vi "Test Executive.vi"(11 "Module Config":T30={"Name"="Test Executive", "Parent Q"=refnum, "Is Child?"=FALSE, "Index"=0, "Dirs"={"Root"=path "C:/MTE", "Config"=path "C:/MTE/Config", "Logs"=path "C:/MTE/Logs", "Reports"=path "C:/ATE/Reports", "App Data"=path "C:/ProgramData/Test Executive"}, "Simulate"=FALSE, "SimCtrl"=refnum}) -> ()   [LabVIEW 2018] (continued)
                  n74 = To More Generic Class(target class=w219, reference=w220) -> (generic class reference=w218:refnum<vi>)
                  n75 = To More Generic Class(target class=w219, reference=w223) -> (generic class reference=w224:refnum<vi>)
                  n76 = To More Generic Class(target class=w219, reference=w221) -> (generic class reference=w222:refnum<vi>)
                  n77 = Build Array (concatenate)(w225, w224, w222, w218) -> (w226:refnum<vi>[])
                }
                frame 99, Default {
                  # "Done"
                }
              }
            }
            n78 = Unbundle By Name(w208) -> ("CtrlStates"=w210:refnum<class "Class.SaveCtrls.lvclass">, "Cfg.Name"=w212:string, "Cfg.Dirs.App Data"=w211:path)
            n79 = call-dynamic "Class.SaveCtrls.InitLoadRestore.vi"("Ctrl Array"=w209, "Module Data Dir"=w211, "Module Name"=w212, "CtrlStates In"=w210) -> ("CtrlStates"=w207:refnum<class "Class.SaveCtrls.lvclass">)  [unwired: 6 in, 1 out]
          }
          frame #5 {
            w229 = T17[] []  # RptCfg
            w230 = T58[] []  # Subscr
            w232 = FALSE  # TestCanceled
            w233 = T20 {"DispDetails"=FALSE, "NotResetSN"=FALSE, "NotValOper"=FALSE, "NotValSN"=FALSE, "DisResults"=FALSE, "StaModule"=FALSE, "EditEQ"=FALSE, "ClrWarn"=FALSE, "ClrErr"=FALSE, "ViewCfg"=FALSE, "SetOpts"=FALSE, "ContOnErr"=FALSE, "ContOnFail"=FALSE, "DisMetrics"=FALSE, "SelSeq"=FALSE, "GenRpt"=FALSE, "DisStartWithSN"=FALSE, "Auto Repeat Seq En"=FALSE, "DataDirEn"=FALSE, "SNRouteCk"=FALSE}  # Opts
            w238 = path ""  # UUT Dir
            w239 = -1.0  # Repeat(s)
            w241 = T69 {"Limits"=variant, "Limit File"="", "Limit Ver"="", "RsltCodes"=variant, "Rslt Code File"="", "Rslt Code Ver"="", "Default Seq"=0, "FaultPrefix"=0, "UUTRoutes"=[], "DisableRouteCk"=FALSE, "StaVer"=0, "SN Valid"=FALSE, "ReqVars"=FALSE, "Product"="", "ProcessStep"="", "FileSyncMaster"=path "", "CmtPrmpt"=FALSE}  # Lists
            w243 = T50 {"Position"="", "Result"={"Result"=enum."Pass", "Code"=0, "Description"=""}, "Measurements"={"Measurement"=[]}, "UUTInfo"={"Product"="", "Desc"="", "PN"="", "SN"="", "Lot"="", "DateCode"="", "AltID"="", "Revision"="", "Properties"={"Property"=[]}}}  # RptUUT
            w242 = T70 {"#attributes"={"Version"="MTE_2.0.0"}, "Facility"={"Name"="", "Location"=""}, "Station"={"Name"="", "PN"="", "SN"="", "Rev"="", "PC Name"="", "Location"="", "HW_Config"={"HW_Item"=[]}, "SW_Config"={"SW_Item"=[]}}, "Test Run"={"Operator"="", "Start Time"=timestamp(0 s since 1904-01-01), "Duration(s)"=0.0, "Mode"="", "Comment"="", "ProcessStep"=""}, "Test Sequence"={"Name"="", "Config"={"Config_Item"=[]}}}  # RptHdr
            w244 = cluster{"FileObjs":T29[], "Meas":T38[]} {"FileObjs"=[], "Meas"=[{"Cnt"=0, "Step"="", "Category"="", "Name"="", "Value"="", "Units"="", "LimType"="", "LL"="", "UL"="", "Status"=0, "Code"=0, "Desc"="", "Time"=timestamp(0 s since 1904-01-01)}]}  # Data
            w245 = T72 {"Level"=0, "Cnts"=[], "Step"="", "Cntr"=0}  # SectCtr
            w246 = errorcluster {"status"=FALSE, "code"=0, "source"=""}  # ResultError
            w247 = FALSE  # DisableResults
            w231 = variant  # SW_Vers
            n80 = call <vilib>:"Q.Enqueue Task.vi"("Top of Q"=TRUE, "Task Name"="Test Metrics - Load", "Q In"=w236) -> ("Q Out"=w237:refnum<queue>)  [unwired: 7 in, 1 out]
            n81 = call <vilib>:"Q.Enqueue Seq.vi"("Top of Q"=TRUE, "Seq Task Name"="Init Controls", "Q In"=w237) -> ()  [unwired: 7 in, 2 out]
            "Failing Status" <- "Failing" ("Failing Status")
          }
          frame #6 {
            # "Setup Menu"
            n82 = Current VI's Menubar() -> (w250:refnum<k9>)
            n83 = while {
              tunnel: w250 -> [w251]
              i -> [w253]
              stop <- w252 stop-if-true
              n84 = case shown="1" w253 {
                tunnel: [_ _ _ _ _ _ _ _ _ _ TRUE] -> w252
                tunnel: w251 -> [w259 w260 w265 w268 w271 w274 w277 w280 w284 w288 w290]
                frame 0 {
                  w256 = "Data"
                  n85 = Insert Menu Items(4:"Config" ("menu tag"), 7:w256, 8:w256, 9:w259) -> (0:w254:errorcluster, 3:w257:refnum<k9>)  [unwired: 2 in, 1 out]
                  n86 = call <vilib>:"Menu.Enable Item.vi"("error in"=w254, "Enable"=FALSE, "Tag"=w256, "Menu Ref"=w257) -> ()  [unwired: 6 in, 2 out]
                }
                frame 1 {
                  w262 = "Route Check"
                  n87 = Insert Menu Items(4:"Config" ("menu tag"), 7:w262, 8:w262, 9:w260) -> ()  [unwired: 2 in, 3 out]
                }
                frame 2 {
                  w264 = "Test Executive"
                  n88 = Insert Menu Items(5:"Config" ("menu tag"), 7:w264, 8:w264, 9:w265) -> ()  [unwired: 2 in, 3 out]
                }
                frame 3 {
                  w267 = "Local Station"
                  n89 = Insert Menu Items(5:"Config" ("menu tag"), 7:w267, 8:w267, 9:w268) -> ()  [unwired: 2 in, 3 out]
                }
                frame 4 {
                  w270 = "File Sync"
                  n90 = Insert Menu Items(5:"Config" ("menu tag"), 7:w270, 8:w270, 9:w271) -> ()  [unwired: 2 in, 3 out]
                }
                frame 5 {
                  w273 = "File Rotate"
                  n91 = Insert Menu Items(5:"Config" ("menu tag"), 7:w273, 8:w273, 9:w274) -> ()  [unwired: 2 in, 3 out]
                }
                frame 6 {
                  w276 = "Test Reports"
                  n92 = Insert Menu Items(5:"Config" ("menu tag"), 7:w276, 8:w276, 9:w277) -> ()  [unwired: 2 in, 3 out]
                }
                frame 7 {
                  w279 = "Mode Manager"
                  n93 = Insert Menu Items(5:"Config" ("menu tag"), 7:w279, 8:w279, 9:w280) -> ()  [unwired: 2 in, 3 out]
                }
                frame 8 {
                  n94 = Insert Menu Items(5:"Config" ("menu tag"), 7:"Config_Config Folder", 8:"Open Config Folder", 9:w284) -> ()  [unwired: 2 in, 3 out]
                }
                frame 9 {
                  n95 = Insert Menu Items(5:"Config" ("menu tag"), 7:"Config_Test Sequence Folder", 8:"Open Test Sequence Folder", 9:w288) -> ()  [unwired: 2 in, 3 out]
                }
                frame Default {
                  n96 = call <vilib>:"Menu.Enable Item.vi"("Enable"=FALSE, "Tag"="Config" ("menu tag"), "Menu Ref"=w290) -> ()  [unwired: 7 in, 2 out]
                }
              }
            }
          }
          frame #7 {
            # "Setup Config Files - if they do not exist"
            n97 = Unbundle By Name(w293) -> ("Cfg.Dirs"=→"Cfg.Dirs":T27, "Cfg.Dirs.Root"=w297:path)
            n98 = local read "Title"() -> (w295:string)
            n99 = call "TestExec.Init Config Files at Launch.vi"("Station Name"=w295, "Working Dir"=w297) -> ("error out"=w296:errorcluster)  [unwired: 9 in]
            n100 = call <vilib>:"Clear Errors.vi"("error in (no error)"=w296) -> ()  [unwired: 5 in, 2 out]
          }
          frame #8 {
            # "If config, add remote listener\nUse 'Remote' as Cmd and individual tasks\nUse 'Data' as cmd for events\nUse 'Task' Subscribe to subscribe to data events\n\nSupport:\n  Connection Status Updates\n  Commands:\n     Test Start(SN, Nest, Sequence) \n         Reply: ACK or NAK\n         If Seq is missing will run current sequence\n     Test State()\n         Reply: ACK, State\n    Test Abort\n         Reply: ACK, 1 if aborted, 0 if nothjing to abort\n \n\n Subscribe(EventName)\n     Subscribe to events:\n         Name: Data\n         TestDone: Result, Code, Desc\n         TestStart:\n         Error: Code, Desc\n\nProtocol:\n1st 2 byts is message length\nRest is tab delimited string\nAlways replay with ACK or NAK + description"
            n101 = Unbundle By Name(w301) -> ()  [unwired: 1 out]
            n102 = control-ref of="Remote"() -> (w299:refnum<vi>)
            n103 = property class="Bool (strict)"(reference=w299, "Visible"=FALSE) -> ()  [unwired: 1 in, 2 out]
            "Remote" <- FALSE ("Remote")
          }
          frame #9 {
            n104 = vi-ref "TestExec.Run Executable and Rtn.vi"() -> (w307:refnum<vi>)
            n105 = vi-ref "TestExec.Run Executable and Parse Results V2vi.vi"() -> (w308:refnum<vi>)
            n106 = call <vilib>:"File.Rotate.Manager - Reference.vi"() -> ("VI Refnum"=w306:refnum<vi>)  [unwired: 11 in]
            n107 = invoke on="RunExe Sub Panel" class="SubPnl" method="Insert VI"("VI Ref"=w307) -> (error out=w304:errorcluster)  [unwired: 3 in, 3 out]
            n108 = invoke on="RunUtil Sub Panel" class="SubPnl" method="Insert VI"("VI Ref"=w308) -> (error out=w305:errorcluster)  [unwired: 3 in, 3 out]
            n109 = invoke on="Sub Panel - FileRotation" class="SubPnl" method="Insert VI"("VI Ref"=w306) -> (error out=w303:errorcluster)  [unwired: 3 in, 3 out]
            n110 = Merge Errors(w305, w304, w303) -> (w302:errorcluster)
            n111 = call <vilib>:"Clear Errors.vi"("error in (no error)"=w302) -> ()  [unwired: 5 in, 2 out]
          }
          frame #10 {
            # "Startup Scripts"
            n112 = Unbundle By Name(w314) -> ("Cfg.Dirs.Config"=w312:path)
            n113 = Build Path(base path=w312, name or relative path="StartUp") -> (appended path=w311:path)
            n114 = call <vilib>:"File.Check if File or Folder Exists.vi"("Path"=w311) -> ("Exists"=w310:bool, "Dup Path"=w309:path)  [unwired: 6 in, 3 out]
            n115 = case shown="True" w310 {
              tunnel: w309 -> [_ w315]
              frame False {
              }
              frame True {
                n116 = stacked-sequence {
                  seq-local: [w319 _ _] -> [_ _ w328]
                  seq-local: [w318 _ _] -> [_ _ w327]
                  seq-local: [w317 _ _] -> [_ _ w326]
                  tunnel: w315 -> [_ w324 _]
                  tunnel: [_ w322 _] -> _
                  tunnel: [w316 _ _] -> _
                  tunnel: [_ _ w325] -> _
                  frame #0 {
                    n117 = control-ref of="Status"() -> (w321:refnum<vi>)
                    n118 = call "String.Notification Message - Set Text Box State.vi"("Message"="Running initialize scripts, Please Wait.", "TxtBoxRef"=w321) -> ("error out"=w316:errorcluster, "OldColor"=w317:u32, "OldValue"=w318:string, "RefOut"=w319:refnum<vi>)  [unwired: 6 in]
                  }
                  frame #1 {
                    w323 = TRUE ("Wait til Complete")
                    n119 = call "CmdExe.Run Multiple Utilities.vi"("Show Cmd Window"=w323, "Wait til Complete"=w323, "Util Folder"=w324) -> ("error out"=w322:errorcluster)  [unwired: 7 in, 1 out]
                  }
                  frame #2 {
                    n120 = call "String.Notification Message - Set Text Box State.vi"("NewColor"=w326, "Message"=w327, "TxtBoxRef"=w328) -> ("error out"=w325:errorcluster)  [unwired: 5 in, 3 out]
                  }
                }
              }
            }
          }
        }
        n121 = Bundle By Name(cluster=w83, "CtrlStates"=w80) -> (w84:T33)
        n122 = Bundle("Lnch"=w77, "SeqTimer"=w87, "TimeOut(s)"=w86, "ModeMgr"=w85, "CfgFilePaths"=w82, "Data Dirs"=w81, "StaApp"=w76, "App"=w79, "Sequences"=w72, "PreTestCk"=w71, "Seq"=w70, "SeqMgr"=w69, "Health"=w68, "ResultState"=w67, "SW_Vers"=w66, "Repeat(s)"=w65, "DisableResults"=w64, "SectCtr"=w63, "Data"=w62, "ResultError"=w61, "RptHdr"=w60, "RptUUT"=w59, "Lists"=w57, "TestCanceled"=w56, "Opts"=w55, "UUT Dir"=w54, "Funct"=w53, "StaNotify"=w52, "Subscr"=w51, "Sync"=w50, "RptCfg"=w49) -> (w75:T73)  [unwired: 1 in]
        n123 = Bundle By Name(cluster=w75, "StaApp"=w73) -> (w74:T73)
      }
      frame "Reset" {
        # "Reinit Local Data"
        n124 = stacked-sequence {
          tunnel: w338 -> [_ _ w375 _ w413 _]
          tunnel: w337 -> [_ _ _ _ w414 _]
          tunnel: w336 -> [_ w371 w378 _ w423 _]
          tunnel: w335 -> [w345 w368 _ _ _ w437]
          tunnel: [_ w361 _ _ _ _] -> w331
          tunnel: [_ w364 _ _ _ _] -> w330
          frame #0 {
            w349 = u32 16448250
            w356 = T36."Enabled" ("Disabled")
            w340 = 0
            # "*** Indicators ***"
            # "**** Tabs ***"
            # "*** Status ***"
            # "Init Controls"
            n125 = Unbundle By Name(w345) -> ("Log"=w346:refnum<class "Event Notification.lvclass">)
            n126 = invoke on="SN Rslt" class="Str" method="Reinit To Default"() -> ()  [unwired: 3 in, 3 out]
            n127 = invoke on="Comment" class="Str" method="Reinit To Default"() -> ()  [unwired: 3 in, 3 out]
            n128 = property on="Status" class="Str"("Text.BGColor"=u32 13816530) -> ()  [unwired: 2 in, 2 out]
            n129 = local write "SN"("") -> ()
            n130 = call <vilib>:"Event Notification.Status Message.vi"("Log"=TRUE, "Message"="Reset - Initializing", "Event Notification in"=w346) -> ()  [unwired: 9 in]
            n131 = local write "Test Ctrl Tab"(enum32{"Idle", "Running", "Completed"}."Idle" ("Test Ctrl Tab")) -> ()
            n132 = property on="SN" class="Str"("DisabledEnum"=w356) -> ()  [unwired: 2 in, 2 out]
            n133 = local write "Main Tab"(w340) -> ()
            n134 = local write "Test Status Tab"(w340) -> ()
            n135 = property on="Operator" class="Str"("DisabledEnum"=w356) -> ()  [unwired: 2 in, 2 out]
            n136 = local write "Mode"(0) -> ()
            n137 = local write "Funct Tab"(w340) -> ()
            n138 = local write "Test Status Tab Sel"(w340) -> ()
            n139 = property on="Sequence" class="Ring (strict)"("DisabledEnum"=T36."Enabled" ("Disabled")) -> ()  [unwired: 2 in, 2 out]
            n140 = property on="Start" class="Bool"("DisabledEnum"=T36."Enabled" ("Disabled")) -> ()  [unwired: 2 in, 2 out]
            n141 = local write "Test State"(enum32{"Idle", "Running", "Completed"}."Idle" ("Test State")) -> ()
            n142 = property on="Repeat Notificaiton" class="Str"("Visible"=FALSE) -> ()  [unwired: 2 in, 2 out]
            n143 = property class="App"() -> ("App.UserName"=w353:string)  [unwired: 2 in, 2 out]
            n144 = property on="Abort Cnt" class="DigNum (strict)"("NumText.BGColor"=u32 16448250) -> ()  [unwired: 2 in, 2 out]
            n145 = property on="Fail Cnt" class="DigNum (strict)"("NumText.BGColor"=w349) -> ()  [unwired: 2 in, 2 out]
            n146 = property on="Error Cnt" class="DigNum (strict)"("NumText.BGColor"=w349) -> ()  [unwired: 2 in, 2 out]
            n147 = property on="Yield%" class="DigNum (strict)"("NumText.BGColor"=w349) -> ()  [unwired: 2 in, 2 out]
            n148 = invoke on="Abort Flag" class="Bool (strict)" method="Reinit To Default"() -> ()  [unwired: 3 in, 3 out]
            n149 = property on="Prompt2_OK" class="Bool"("DisabledEnum"=T36."Enabled" ("Disabled")) -> ()  [unwired: 2 in, 2 out]
            n150 = property on="Kill AutoLnch" class="Bool"("Visible"=FALSE) -> ()  [unwired: 2 in, 2 out]
            n151 = local write "Operator"(w353) -> ()
            n152 = local write "PLC Enable"(TRUE ("PLC Enable")) -> ()
            n153 = invoke on="Abort Cnt" class="DigNum (strict)" method="Reinit To Default"() -> ()  [unwired: 3 in, 3 out]
          }
          frame #1 {
            w363 = T74 -5201 items=["No Error"=0, "Abort"=-2, "Misc"=-5000, "Fixture Error"=-5100, "File IO - General"=-5200, "FIle IO - Config Error"=-5201, "Instrument - General"=-5300, "Instrument - Serial Com"=-5301, "Instrument - Camera"=-5302, "Instrument - PS"=-5303, "Instrument - Oscilloscope"=-5304, "Instrument - Function Gen"=-5305, "Instrument - Load"=-5306, "Instrument - Meter"=-5307, "Instrument - Power Control"=-5308, "Instrument - Motion"=-5309, "Instrument - RF"=-5310, "System Exe"=-5400, "Image Processing"=-5500, "Communication"=-5600, "Script - Syntax Error"=-6000, "Script - Invalid Name or Param"=-6100, "Script - Timeout"=-6200, "Invalid Data"=-6300, "FW Update Error"=-6500] ("Std Code")
            w373 = FALSE ("Repeat Seq")
            # "Lock Controls until after initialization is completed"
            n154 = invoke on="OperNo" class="Bool" method="Reinit To Default"() -> ()  [unwired: 3 in, 3 out]
            n155 = invoke on="OperOK" class="Bool" method="Reinit To Default"() -> ()  [unwired: 3 in, 3 out]
            n156 = invoke on="Prompt2_OK" class="Bool" method="Reinit To Default"() -> ()  [unwired: 3 in, 3 out]
            n157 = Unbundle By Name(w368) -> ("Cfg.Dirs.Config"=w367:path)
            n158 = Unbundle By Name(w371) -> ("Sync"=w370:refnum<class "File.Sync.lvclass">)
            n159 = Build Path(base path=w367, name or relative path="File Sync Config.csv") -> (appended path=w365:path)
            n160 = property on="Start" class="Bool"("DisabledEnum"=T36."Disabled and Grayed Out" ("Disabled")) -> ()  [unwired: 2 in, 2 out]
            n161 = call-dynamic "FileSync.Read Config.vi"("Dialog"=FALSE, "Config File"=w365, "File.Sync in"=w370) -> ("error out"=w360:errorcluster, "File.Sync out"=w361:refnum<class "File.Sync.lvclass">)  [unwired: 5 in, 2 out]
            n162 = local write "Repeat Seq"(w373) -> ()
            n163 = property on="Repeat Seq" class="Bool (strict)"("Visible"=w373) -> ()  [unwired: 2 in, 2 out]
            n164 = property on="RepeatInt(s)" class="DigNum (strict)"("Visible"=w373) -> ()  [unwired: 2 in, 2 out]
            n165 = call "Error.Set-Change Error Info.vi"("Std Code"=w363, "error in"=w360, "Description"="Error reading Sync File Config. ") -> ("error out"=w364:errorcluster)  [unwired: 8 in]
            "PLC Running" <- FALSE ("PLC Running")
          }
          frame #2 {
            n166 = Unbundle By Name(w378) -> ("Lnch"=w377:bool, "App.Child Modules"=w376:cluster{"VI Ref":refnum<vi>, "Name":string}[])
            n167 = case shown="False" w377 {
              tunnel: w376 -> [w379 _]
              tunnel: w375 -> [_ _]
              frame False {
                # "Reset Child Modules"
                n168 = for {
                  tunnel: w379 -> [w384] mode=indexing
                  tunnel: [w381] -> _ mode=indexing
                  n169 = Unbundle By Name(w384) -> ("Name"=w383:string)
                  n170 = call <vilib>:"Q.Enqueue Item.vi"("Top of Q"=TRUE, "Q Name"=w383, "Cmd"="Reset") -> ("error out"=w381:errorcluster)  [unwired: 7 in, 1 out]
                }
              }
              frame True {
                # "Do not reset at launch.\nThey are already reset"
              }
            }
          }
          frame #3 {
            w386 = FALSE ("Comment At End")
            w385 = T36."Disabled and Grayed Out" ("Disabled")
            w393 = T36."Disabled and Grayed Out" ("Disabled")
            w395 = T36."Enabled" ("Disabled")
            w401 = FALSE ("Blinking")
            w389 = 0.0 ("Progress")
            n171 = invoke on="Enable File Sync" class="Bool (strict)" method="Reinit To Default"() -> ()  [unwired: 3 in, 3 out]
            n172 = property on="Test Running" class="Bool (strict)"("Blinking"=w401) -> ()  [unwired: 2 in, 2 out]
            n173 = property on="Operator" class="Str"("DisabledEnum"=w395, "Text.BGColor"=u32 16448250) -> ()  [unwired: 2 in, 2 out]
            n174 = property on="SN" class="Str"("DisabledEnum"=w395, "Text.BGColor"=u32 16383928) -> ()  [unwired: 2 in, 2 out]
            n175 = invoke on="Duration(HH:MM:SS)" class="Str" method="Reinit To Default"() -> ()  [unwired: 3 in, 3 out]
            n176 = property on="SN" class="Str"("Key Focus"=TRUE) -> ()  [unwired: 2 in, 2 out]
            n177 = property on="Test Status Tab" class="TabCtl (strict)"("Tabs Visible?"=FALSE) -> ()  [unwired: 2 in, 2 out]
            n178 = invoke on="Filter" class="Str" method="Reinit To Default"() -> ()  [unwired: 3 in, 3 out]
            n179 = Get Date/Time In Seconds() -> (seconds since 1Jan1904=→"End Time" →"Start Time":timestamp)
            n180 = property on="OperOK" class="Bool"("DisabledEnum"=w393) -> ()  [unwired: 2 in, 2 out]
            n181 = property on="OperNo" class="Bool"("DisabledEnum"=w393) -> ()  [unwired: 2 in, 2 out]
            n182 = property on="Results Table" class="Arr (strict)"("Index Values"=u32[] [0]) -> ()  [unwired: 2 in, 2 out]
            n183 = property on="Inc Step" class="Bool"("DisabledEnum"=T36."Disabled and Grayed Out" ("Disabled")) -> ()  [unwired: 2 in, 2 out]
            n184 = property on="Step Run" class="Bool"("DisabledEnum"=T36."Disabled and Grayed Out" ("Disabled")) -> ()  [unwired: 2 in, 2 out]
            n185 = call "Time.Secs to H_M_S Duration.vi"("Total Secs"=w389) -> ("Duration(HH:MM:SS)"=→"Duration(HH:MM:SS)":string)  [unwired: 10 in]
            n186 = property on="Pause" class="Bool (strict)"("Value"=FALSE ("Single Step")) -> ()  [unwired: 2 in, 2 out]
            n187 = property on="PersistCmt" class="Bool (strict)"("DisabledEnum"=w385, "Value"=w386) -> ()  [unwired: 2 in, 2 out]
            n188 = property on="Comment At End" class="Bool (strict)"("DisabledEnum"=w385, "Value"=w386) -> ()  [unwired: 2 in, 2 out]
            "Result Status" <- T2 {"State"=enum."None", "Code"=0, "Description"=""} ("Result")
            "Duration(s)" <- w389
            "Progress" <- w389
            "UUT SN Status" <- "Enter Operator and SN then click Start." ("UUT SN Status")
            "Test Running" <- w401
            "FileSyncActive" <- FALSE ("FileSyncActive")
          }
          frame #4 {
            # "Queue Initialization Tasks"
            n189 = Flush Queue(queue=w413, error in (no error)=w414) -> (queue out=w415:refnum<queue>, error out=w416:errorcluster)  [unwired: 1 out]
            n190 = call <vilib>:"Scheduler.Clear-Reset.vi"("error in"=w416, "Q In"=w415) -> ("Q Out"=w405:refnum<queue>)  [unwired: 8 in, 1 out]
            n191 = Unbundle By Name(w423) -> ("Lnch"=w424:bool)
            n192 = To Variant(anything=TRUE) -> (Variant=w411:variant)
            n193 = call <vilib>:"Q.Enqueue App.vi"("Data1"=w411, "Task Name"="Lock Test Controls", "Q In"=w405) -> ("Q Out"=w409:refnum<queue>)  [unwired: 7 in, 1 out]
            n194 = To Variant(anything=TestExec.Health_State_Command."Clear All" ("Health State Cmd")) -> (Variant=w407:variant)
            n195 = call <vilib>:"Q.Enqueue App.vi"("Data1"=w407, "Task Name"="Health Status", "Q In"=w409) -> ("Q Out"=w404:refnum<queue>)  [unwired: 7 in, 1 out]
            n196 = for {
              shift-right: [w435] -> w426
              shift-left: w404 -> [w434]
              tunnel: string[] ["Init Temp Dir", "Config - Read", "Config - Set File Sync", "Config - Set Reports", "Maint - Scheduler"] -> [w433] mode=indexing
              n197 = call <vilib>:"Q.Enqueue Task.vi"("Task Name"=w433, "Q In"=w434) -> ("Q Out"=w435:refnum<queue>)  [unwired: 8 in, 1 out]
            }
            n198 = call <vilib>:"Q.Enqueue Seq.vi"("Seq Task Name"="Test Reset", "Q In"=w426) -> ("Q Out"=w417:refnum<queue>)  [unwired: 8 in, 1 out]
            n199 = case shown="True" w424 {
              tunnel: w417 -> [w429 w432]
              tunnel: [w429 w431] -> w422
              tunnel: "Simulate Fwd" ("Sched Name") -> [_ w430]
              frame False {
              }
              frame True {
                n200 = call <vilib>:"Q.Enqueue App.vi"("Task Name"=w430, "Q In"=w432) -> ("Q Out"=w431:refnum<queue>)  [unwired: 8 in, 1 out]
              }
            }
            n201 = call <vilib>:"Q.Enqueue App.vi"("Task Name"="Initialization Done", "Q In"=w422) -> ("Q Out"=w420:refnum<queue>)  [unwired: 8 in, 1 out]
            n202 = call <vilib>:"Q.Enqueue App.vi"("Top of Q"=TRUE, "Task Name"="Set Logging Level", "Q In"=w420) -> ()  [unwired: 7 in, 2 out]
          }
          frame #5 {
            n203 = Unbundle By Name(w437) -> ("Cfg.Dirs.Config"=w438:path)
            n204 = call "TestExec.Config, Get Station SW Module Info.vi"("Path"=path "C:/MTE/Test Executive/Config") -> ("error out"=w443:errorcluster, "Sta Exe Path"=w442:path)  [unwired: 7 in, 2 out]
            n205 = Empty String/Path?(string/path=w442) -> (empty?=w441:bool)
            n206 = case shown="False" w441 {
              tunnel: w443 -> [w452 _]
              tunnel: w442 -> [w450 _]
              tunnel: [w444 _] -> _
              frame False {
                n207 = call <vilib>:"File.Open File or Folder.vi"("Error In"=w452, "Path"=w450) -> ("Error Out"=w451:errorcluster)  [unwired: 9 in]
                n208 = control-ref of="This VI"() -> (w449:refnum<vi>)
                n209 = call <vilib>:"Clear Errors.vi"("error in (no error)"=w451) -> ("error out"=w448:errorcluster)  [unwired: 5 in, 1 out]
                n210 = property class="VI"(reference=w449, error in=w448, "Front Panel.IsFrontmost"=TRUE ("Front Panel Window:Is Frontmost")) -> (error out=w446:errorcluster)  [unwired: 1 out]
                n211 = property on="SN" class="Str"(error in=w446, "Key Focus"=TRUE ("Front Panel Window:Is Frontmost")) -> (error out=w444:errorcluster)  [unwired: 1 in, 1 out]
              }
              frame True {
              }
            }
            n212 = List Folder(path=w438, pattern="Util*.ini") -> (filenames=w436:string[])  [unwired: 2 in, 3 out]
            n213 = property on="Utility INI Config File" class="Ring (strict)"("Strings []"=w436) -> ()  [unwired: 2 in, 2 out]
          }
        }
        n214 = Bundle By Name(cluster=w336, "Lnch"=FALSE ("Test.Running"), "PreTestCk"=T35 {"Oper"={"OK"=FALSE, "Desc"=""}, "SN"={"OK"=FALSE, "Desc"=""}, "NoSN"=FALSE, "DefaultSN"="", "SNErr"=FALSE, "SeqEn"=enum."Enabled"}, "Repeat(s)"=-1.0, "Health.Init"=TRUE ("Test.Running"), "Sync"=w331) -> (w339:T73)
      }
      frame "Task" {
        n215 = case shown="\"SeqCmd\"" w458 {
          selector: w458 -> [w466 _ _ _ _ _ _ _ _ _ _ _ w987 _ _ w1074 _ _ _ _ _ _ _ _ _ _ _ w1499 w1516 _ _ _ _ _ _ _ _ _ _ _ _ _ _ _ _ _ _ _ _ _ w2198 _ _ _ _ w3758 _ _ _ _ _ _ _ _ _ w3925 _ _ _ _ _ _ _ _ _ _ _ _ _ _ _ _ _ w4301]
          tunnel: w462 -> [w471 w517 w555 w566 w600 w623 w857 w885 w894 w934 w978 w982 w994 w1021 w1070 w1072 w1179 w1205 w1213 w1227 w1256 w1263 w1282 w1296 w1306 w1333 w1491 w1503 w1520 w1532 w1539 w1547 w1608 w1655 w1667 w1680 w1684 w1703 w1720 w1757 w1970 w2002 w2023 w2063 w2079 w2107 w2137 w2149 w2183 w2195 w2199 w3689 w3711 w3732 w3746 w3755 w3790 w3819 w3832 w3842 w3852 w3858 w3862 w3869 w3870 w3922 w4018 w4048 w4066 w4070 w4088 w4089 w4109 w4123 w4152 w4177 w4186 w4201 w4228 w4239 w4251 w4272 w4297 w4304]
          tunnel: w461 -> [w464 w518 w556 w567 w596 w624 w859 w884 w891 w916 w963 w980 w990 w1025 w1062 w1078 w1175 w1206 w1210 w1231 w1255 w1260 w1278 w1293 w1304 w1332 w1490 w1501 w1518 w1534 w1538 w1546 w1612 w1654 w1664 w1676 w1682 w1701 w1737 w1758 w1972 w1999 w2018 w2061 w2077 w2109 w2136 w2152 w2175 w2194 w2201 w3696 w3707 w3738 w3750 w3763 w3789 w3822 w3831 w3841 w3851 w3857 w3861 w3868 w3875 w3928 w4021 w4049 w4065 w4069 w4085 w4095 w4101 w4126 w4155 w4179 w4187 w4203 w4227 w4235 w4261 w4268 w4296 w4303]
          tunnel: [w471 w517 w555 w566 w600 w618 w857 w885 w894 w934 w978 w982 w994 w1021 w1070 w1072 w1179 w1205 w1213 w1227 w1256 w1263 w1282 w1296 w1306 w1333 w1491 w1503 w1520 w1532 w1539 w1547 w1608 w1655 w1667 w1680 w1684 w1703 w1720 w1757 w1970 w2002 w2023 w2063 w2079 w2107 w2137 w2149 w2183 w2195 w2199 w3689 w3711 w3732 w3746 w3755 w3790 w3819 w3832 w3842 w3852 w3858 w3862 w3869 w3870 w3922 w4018 w4048 w4066 w4070 w4088 w4089 w4109 w4123 w4152 w4177 w4186 w4201 w4228 w4239 w4251 w4272 w4297 w4304] -> w460
          tunnel: [w465 w525 w559 w573 w596 w625 w859 w884 w892 w933 w977 w980 w993 w1026 w1071 w1076 w1174 w1206 w1209 w1228 w1254 w1259 w1278 w1292 w1322 w1331 w1490 w1501 w1518 w1534 w1538 w1554 w1614 w1653 w1664 w1675 w1683 w1702 w1738 w1758 w1972 w1998 w2017 w2062 w2078 w2109 w2135 w2152 w2181 w2194 w2200 w3693 w3707 w3723 w3747 w3757 w3789 w3822 w3830 w3840 w3851 w3857 w3861 w3868 w3872 w3924 w4019 w4049 w4065 w4069 w4085 w4095 w4100 w4126 w4155 w4179 w4187 w4203 w4227 w4235 w4257 w4269 w4296 w4303] -> w459
          tunnel: w457 -> [w470 w527 w560 w575 w610 _ w873 _ _ w929 w976 _ w992 _ _ _ _ _ _ w1222 _ _ w1281 w1295 _ _ _ _ _ _ _ _ _ _ _ _ _ w1686 w1726 _ w1962 w2001 w2006 w2054 w2072 _ w2134 _ w2182 _ w2207 w3697 w3714 w3739 w3751 w3765 _ _ w3829 w3839 _ _ _ _ w3878 w3927 _ _ _ _ _ w4094 w4108 w4130 _ _ _ _ _ _ w4260 w4271 w4293 w4307]
          tunnel: w456 -> [w463 _ _ w563 _ w621 _ _ _ _ _ _ _ w1007 _ w1077 w1172 _ w1212 w1224 _ w1262 w1268 _ _ _ _ _ _ _ _ w1548 w1613 w1651 w1661 w1672 _ w1689 w1728 _ _ _ w2012 w2058 w2074 _ w2130 _ w2178 _ w2196 _ _ _ _ _ _ _ w3824 w3836 _ _ _ _ w3873 w3923 w4020 _ _ _ _ _ _ _ w4136 w4167 w4180 w4191 _ w4236 _ _ w4294 _]
          tunnel: w455 -> [_ _ _ _ _ _ _ _ _ _ _ _ _ _ _ _ _ _ _ _ _ _ _ _ _ _ _ _ _ _ _ _ _ _ _ _ _ _ _ _ _ _ _ _ _ _ _ _ _ _ _ _ _ _ _ _ _ _ _ _ _ _ _ _ _ _ _ _ _ _ _ _ _ _ _ _ _ _ _ _ _ _ w4292 w4305]
          tunnel: w454 -> [_ _ _ _ _ _ _ _ _ _ _ _ _ _ _ _ _ _ _ _ _ _ _ _ _ _ _ _ _ _ _ _ _ _ _ _ _ _ _ _ _ _ _ _ _ _ _ _ _ _ w2204 _ _ _ _ _ _ _ _ _ _ _ _ _ _ w3926 _ _ _ _ _ _ _ _ _ _ _ _ _ _ _ _ _ w4306]
          tunnel: [_ _ _ _ _ w620 _ _ _ w923 w970 _ w989 w1013 _ w1073 _ _ _ _ _ _ _ _ _ _ _ _ _ _ _ w1545 w1611 _ _ _ _ _ w1723 w1756 w1963 _ w2003 _ _ w2100 _ w2167 _ _ w2197 _ w3700 _ _ w3760 _ _ _ _ _ _ _ _ _ _ _ _ _ w4068 _ _ _ _ _ _ _ _ _ _ w4258 _ _ w4298] -> w453
          frame "Add_TimeLog" {
            # "TimeLog(Name,[Category])\nThis is used for characterizing and debugging test times. \nCreates a Numeric Data item with the value = time since the test start.\nIf Category is empty, the category will be \"TimeLog\"\nCreates a variable with the logged time in seconds.  This makes the time available to the script."
            n216 = Variant To Data(type=string[] [], Variant=w470) -> (data=w467:string[], error out=w468:errorcluster)  [unwired: 1 in]
            n217 = case shown="Error" w468 {
              selector: w468 -> [_ w515]
              tunnel: w466 -> [_ w512]
              tunnel: [_ w510] -> _
              tunnel: w467 -> [w506 _]
              tunnel: w464 -> [w478 w509]
              tunnel: [w505 w509] -> w465
              tunnel: w463 -> [w503 _]
              frame No Error {
                w507 = T39 0 items=["LOG", "PASS", "FAIL", "ERROR"] ("Status")
                n218 = local read "Start Time"() -> (w483:timestamp)
                n219 = Index Array(array=w506) -> (element #1=w490:string, element #2=w486:string)  [unwired: 2 in]
                n220 = Get Date/Time In Seconds() -> (seconds since 1Jan1904=w482:timestamp)
                n221 = call <vilib>:"Trim Whitespace.vi"("string"=w486) -> ("trimmed string"=w488:string)  [unwired: 1 in]
                n222 = Subtract(x=w482, y=w483) -> (x-y=w474:dbl)
                n223 = Empty String/Path?(string/path=w488) -> (empty?=w487:bool)
                n224 = Format Into String(format string="%#.3f", w474) -> (resulting string=w472:string)  [unwired: 2 in, 1 out]
                n225 = call <vilib>:"Q.Enqueue Task.vi"("Top of Q"=TRUE, "Task Name"="Update Result Table", "Q In"=w503) -> ()  [unwired: 7 in, 2 out]
                n226 = Select(t="TimeLog", s=w487, f=w486) -> (s? t:f=w484:string)
                n227 = Unbundle By Name(w478) -> ("ResultState"=w502:T63, "SectCtr"=w496:T72, "Data.Meas"=w508:T38[])
                n228 = Bundle By Name(cluster=T38 {"Cnt"=0, "Step"="", "Category"="", "Name"="", "Value"="", "Units"="", "LimType"="", "LL"="", "UL"="", "Status"=0, "Code"=0, "Desc"="", "Time"=timestamp(0 s since 1904-01-01)} ("Meas"), "Category"=w484, "Name"=w490, "Value"=w472, "Units"="Secs", "Status"=w507) -> (w492:T38)
                n229 = call "Step Counter.Step Count Controller.vi"("Step Action"=Step_Counter.Action."Data +", "Step State"=w496) -> ("Step"=w499:string, "Step State Out"=w495:T72, "Cntr"=w497:i32)  [unwired: 7 in]
                n230 = Unbundle By Name(w478) -> ("SeqMgr"=w481:refnum<class "SeqMgr.lvclass">)
                n231 = Build Array("TimeLog", w472) -> (w475:string[])
                n232 = Bundle By Name(cluster=w492, "Step"=w499, "Cnt"=w497) -> (w494:T38)
                n233 = Build Array(w475) -> (w479:string[][])
                n234 = Build Array (concatenate)(w508, w494) -> (w501:T38[])
                n235 = call <vilib>:"SeqMgr.Variables - Add, Replace.vi"("Name, Value"=w479, "SeqMgr in"=w481) -> ("SeqMgr out"=w480:refnum<class "SeqMgr.lvclass">)  [unwired: 8 in, 1 out]
                n236 = call "Result.Measurement, Screen for Fail or Error.vi"("Num"=w501, "ResultState In"=w502) -> ("ResultState Out"=w500:T63)  [unwired: 9 in]
                n237 = Bundle By Name(cluster=w478, "SeqMgr"=w480) -> (w477:T73)
                n238 = Bundle By Name(cluster=w477, "ResultState"=w500, "SectCtr"=w495, "Data.Meas"=w501) -> (w505:T73)
              }
              frame Error {
                n239 = Format Into String(format string="Invalid Data to task %s. Expected 1D string.", w512) -> (resulting string=w511:string)  [unwired: 2 in, 1 out]
                n240 = call "Error.Set-Change Error Info.vi"("error in"=w515, "Description"=w511, "Cust Code(0 = no change)"=-5500 ("Code(0 = no change)")) -> ("error out"=w510:errorcluster)  [unwired: 8 in]
              }
            }
          }
          frame "Client - Sequence Config" {
            # "If name exists, over write.\nElse append."
            # "Client - Sequence Config(2D array of Str: Name, Value)"
            n241 = Variant To Data(type=string[][] [], Variant=w527) -> (data=w524:string[][])  [unwired: 1 in, 1 out]
            n242 = Unbundle By Name(w518) -> ("RptHdr.Test Sequence"=w523:T49)
            n243 = Unbundle By Name(w523) -> ("Config.Config_Item"=w520:cluster{"Name":string, "Value":string}[])
            n244 = for {
              tunnel: w520 -> [w529] mode=indexing
              tunnel: [w528] -> w519 mode=indexing
              n245 = Unbundle By Name(w529) -> ("Name"=w528:string)
            }
            n246 = Unbundle By Name(w517) -> ("Log"=w516:refnum<class "Event Notification.lvclass">)
            n247 = for {
              tunnel: w524 -> [w542] mode=indexing
              shift-right: [w540] -> w522
              shift-left: w520 -> [w541]
              tunnel: w519 -> [w536]
              tunnel: w516 -> [w531]
              n248 = Index Array(array=w542) -> (element #1=w534:string, element #2=w533:string)  [unwired: 2 in]
              n249 = Format Into String(format string="Seq Confg, %s, %s", w534, w533) -> (resulting string=w532:string)  [unwired: 2 in, 1 out]
              n250 = Bundle By Name(cluster=cluster{"Name":string, "Value":string} {"Name"="", "Value"=""} ("Setup"), "Name"=w534, "Value"=w533) -> (w538:cluster{"Name":string, "Value":string})
              n251 = Search 1D Array(1D array=w536, element=w534) -> (index of element=w537:i32)  [unwired: 1 in]
              n252 = call <vilib>:"Event Notification.Status Message.vi"("Level"=Event_Log.Log_Level."Debug0", "Message"=w532, "Event Notification in"=w531) -> ()  [unwired: 9 in]
              n253 = case shown="0, Default" w537 {
                selector: w537 -> [w543 _]
                tunnel: w541 -> [w546 w549]
                tunnel: [w545 w548] -> w540
                tunnel: w538 -> [w544 w547]
                frame 0, Default {
                  n254 = Replace Array Subset(array=w546, new element=w544, index=w543) -> (w545:cluster{"Name":string, "Value":string}[])
                }
                frame -1 {
                  n255 = Build Array (concatenate)(w549, w547) -> (w548:cluster{"Name":string, "Value":string}[])
                }
              }
            }
            n256 = Bundle By Name(cluster=w523, "Config.Config_Item"=w522) -> (w521:T49)
            n257 = Bundle By Name(cluster=w518, "RptHdr.Test Sequence"=w521) -> (w525:T73)
          }
          frame "Client - SetEquipmentList" {
            # "Todo - handle overdue cal notification"
            n258 = Variant To Data(type=T41[] [] ("RptHdrInfo.Station.HW_Config.HW_Item"), Variant=w560) -> (data=w557:T41[])  [unwired: 1 in, 1 out]
            n259 = Unbundle By Name(w555) -> ("Log"=w553:refnum<class "Event Notification.lvclass">)
            n260 = call <vilib>:"Event Notification.Status Message.vi"("Log"=TRUE, "Level"=Event_Log.Log_Level."Debug0", "Message"="Recieved Eq List", "Event Notification in"=w553) -> ()  [unwired: 8 in]
            n261 = call "TestExec.Eq List to Table.vi"("Eq List"=w557) -> ("Table"=→"Equipment List":string[][])
            n262 = Bundle By Name(cluster=w556, "RptHdr.Station.HW_Config.HW_Item"=w557) -> (w559:T73)
          }
          frame "Client - SW Items" {
            # "Client - SW Items(1D array of SW Item)"
            # "If name exists, over write.\nElse append."
            n263 = Unbundle By Name(w567) -> ("RptHdr.Station.SW_Config"=w568:cluster{"SW_Item":T31[]})
            n264 = Unbundle By Name(w568) -> ("SW_Item"=w569:T31[])
            n265 = Variant To Data(type=T31[] [], Variant=w575) -> (data=w572:T31[])  [unwired: 1 in, 1 out]
            n266 = for {
              tunnel: w569 -> [w577] mode=indexing
              tunnel: [w576] -> w570 mode=indexing
              n267 = Unbundle By Name(w577) -> ("Name"=w576:string)
            }
            n268 = Unbundle By Name(w566) -> ("Log"=w565:refnum<class "Event Notification.lvclass">)
            n269 = call <vilib>:"Q.Enqueue Task.vi"("Top of Q"=TRUE, "Task Name"="Maint - SW Version Check", "Q In"=w563) -> ()  [unwired: 7 in, 2 out]
            n270 = for {
              tunnel: w572 -> [w584] mode=indexing
              shift-right: [w587] -> w564
              shift-left: w569 -> [w588]
              tunnel: w570 -> [w585]
              tunnel: w565 -> [w578]
              n271 = Unbundle By Name(w584) -> ("Name"=w582:string, "Version"=w581:string)
              n272 = Format Into String(format string="SW Item: %s, Ver: %s", w582, w581) -> (resulting string=w580:string)  [unwired: 2 in, 1 out]
              n273 = Search 1D Array(1D array=w585, element=w582) -> (index of element=w586:i32)  [unwired: 1 in]
              n274 = call <vilib>:"Event Notification.Status Message.vi"("Level"=Event_Log.Log_Level."Debug0", "Message"=w580, "Event Notification in"=w578) -> ()  [unwired: 9 in]
              n275 = case shown="0, Default" w586 {
                selector: w586 -> [w589 _]
                tunnel: w588 -> [w592 w595]
                tunnel: [w591 w594] -> w587
                tunnel: w584 -> [w590 w593]
                frame 0, Default {
                  n276 = Replace Array Subset(array=w592, new element=w590, index=w589) -> (w591:T31[])
                }
                frame -1 {
                  n277 = Build Array (concatenate)(w595, w593) -> (w594:T31[])
                }
              }
            }
            n278 = Bundle By Name(cluster=w568, "SW_Item"=w564) -> (w571:cluster{"SW_Item":T31[]})
            n279 = local write "SW Items"(w564) -> ()
            n280 = Bundle By Name(cluster=w567, "RptHdr.Station.SW_Config"=w571) -> (w573:T73)
          }
          frame "Data - Open Folder" {
            n281 = Variant To Data(type="", Variant=w610) -> (data=w608:string)  [unwired: 1 in, 1 out]
            n282 = Unbundle By Name(w600) -> ("Cfg.Dirs.Root"=w604:path)
            n283 = Unbundle By Name(w596) -> ("Data Dirs.Station Data"=w598:T23[])
            n284 = Build Path(base path=w604, name or relative path="Sequences" ("section")) -> (appended path=w602:path)
            n285 = Bundle By Name(cluster=T23 {"Name"="Test Sequence Folder", "Path"=path ""} ("Working Dirs"), "Name"="Test Sequence Folder", "Path"=w602) -> (w601:T23)
            n286 = Build Array (concatenate)(w598, w601) -> (w599:T23[])
            n287 = for {
              tunnel: w599 -> [w617] mode=indexing
              tunnel: [w616] -> w607
              tunnel: w608 -> [w614]
              tunnel: [w613] -> w606
              stop <- w613 stop-if-true
              n288 = Unbundle By Name(w617) -> ("Path"=w616:path, "Name"=w615:string)
              n289 = Equal?(x=w615, y=w614) -> (x = y?=w613:bool)
            }
            n290 = case shown="True" w606 {
              tunnel: w607 -> [_ w612]
              tunnel: [_ w611] -> _
              frame False {
              }
              frame True {
                n291 = call <vilib>:"File.Open File or Folder.vi"("Path"=w612) -> ("Error Out"=w611:errorcluster)  [unwired: 10 in]
              }
            }
          }
          frame "Config - Read" {
            n292 = while {
              shift-right: [w631] -> _
              shift-left: "Init" -> [w632]
              shift-right: [w627] -> w625
              shift-left: w624 -> [w634]
              tunnel: w621 -> [w630]
              tunnel: [w628] -> w619 mode=indexing
              shift-right: [w626] -> w618
              shift-left: w623 -> [w633]
              stop <- w629 stop-if-true
              n293 = case shown="\"Init\"" w632 {
                tunnel: w634 -> [w640 w664 w688 w698 w710 w721 w729 w759 w782 w822 w831]
                tunnel: [w644 w665 w689 _ _ _ w733 w760 w797 _ _] -> w628
                tunnel: w633 -> [w638 w668 w695 w700 w707 w723 w732 w754 w783 w826 w838]
                tunnel: ["Station ID" "Facility" "Barcode Input" "Mode" "Route" "Sequences" "Data Dir" "Misc Dirs" "SW Check" "Done" "Done"] -> w631
                tunnel: w630 -> [_ _ _ _ w711 _ w734 _ _ w823 _]
                tunnel: [_ _ _ _ _ _ _ _ _ _ TRUE] -> w629
                tunnel: [w646 w669 w694 w698 w709 w725 w731 w758 w815 w822 w828] -> w627
                tunnel: [w647 w668 w695 w700 w707 w723 w732 w754 w783 w826 w838] -> w626
                frame "Init" {
                  n294 = Unbundle By Name(w638) -> ("Cfg.Dirs.Config"=w659:path)
                  n295 = Unbundle By Name(w638) -> ("Cfg.Dirs.App Data"=w650:path)
                  n296 = Unbundle By Name(w638) -> ("Cfg.Dirs.Config"=w637:path)
                  n297 = Build Path(base path=w650, name or relative path="Working Config.ini") -> (appended path=w648:path)
                  n298 = Build Path(base path=w637, name or relative path="Local Station.ini") -> (appended path=w643:path)
                  n299 = Build Path(base path=w659, name or relative path="Local Station.ini") -> (appended path=w639:path)
                  n300 = call <vilib>:"File.Check if File or Folder Exists.vi"("Path"=w639) -> ("Exists"=w656:bool)  [unwired: 6 in, 4 out]
                  n301 = call "TestExec.Distributed INI Config File Reader.vi"("Additional Config Section Names"=string[] ["AdditionalConfig", "Station"], "Initial Config File Path"=w643, "Output Config Path"=w648) -> ("error out"=w645:errorcluster, "Output Config Path Dup"=w636:path)  [unwired: 6 in, 1 out]
                  n302 = Not(x=w656) -> (.not. x?=w657:bool)
                  n303 = call "TestExec.Read Local Station Get SN From UUT Option.vi"("error in"=w645, "Config File Path"=w636) -> ("error out"=w644:errorcluster, "Default Value"=w641:string, "NotRequired"=w642:bool)  [unwired: 7 in]
                  n304 = call "TestExec.Configure Setup and Dialog - Station.vi"("Dialog"=w657, "SectAddFiles"=string[] ["AdditionalConfig"] ("Sections that List Additional Files"), "Local Station Folder"=w659) -> ("Data Out"=w653:variant)  [unwired: 6 in, 2 out]
                  n305 = call "TestExec.Read File Sync Type Option.vi"("Config File Path"=w636) -> ("Diff(T)/All(F)"=w635:bool)  [unwired: 9 in, 1 out]
                  n306 = Unbundle By Name(w638) -> ("AppData"=w655:refnum<class "Class.AppData.lvclass">)
                  n307 = local write "SyncType"(w635) -> ()
                  n308 = call <vilib>:"ClassAppData.Load_Merge Data.vi"("Data In"=w653, "Class - App Data in"=w655) -> ("Class - App Data out"=w654:refnum<class "Class.AppData.lvclass">)  [unwired: 8 in, 1 out]
                  n309 = Bundle By Name(cluster=w640, "CfgFilePaths.WorkingCfg"=w636, "PreTestCk.NoSN"=w642, "PreTestCk.DefaultSN"=w641) -> (w646:T73)
                  n310 = case shown="False" w642 {
                    tunnel: w641 -> [_ w662]
                    frame False {
                    }
                    frame True {
                      n311 = local write "SN"(w662) -> ()
                    }
                  }
                  n312 = Bundle By Name(cluster=w638, "AppData"=w654) -> (w647:T33)
                }
                frame "Station ID" {
                  # "Get Local Station ID Info"
                  n313 = Unbundle By Name(w664) -> ("CfgFilePaths.WorkingCfg"=w663:path)
                  n314 = Unbundle By Name(w668) -> ("Cfg.Name"=w675:string, "SW Rev.Version"=w674:string, "SW Rev.Description"=w672:string)
                  n315 = call "Config.Read Station Info.vi"("Local Station Config File"=w663) -> ("error out"=w665:errorcluster, "Disable SN Route Ck"=w666:bool, "Station"=w667:T47)  [unwired: 7 in, 1 out]
                  n316 = Bundle By Name(cluster=T31 {"Name"="", "PN"="", "Version"="", "Note"=""} ("Software Items"), "Name"=w675, "Version"=w674, "Note"=w672) -> (w676:T31)
                  n317 = Build Array(w676) -> (w671:T31[])
                  n318 = Unbundle By Name(w667) -> ("Name"=w681:string, "PN"=w680:string, "SN"=w679:string, "Location"=w678:string)
                  n319 = Bundle By Name(cluster=w667, "SW_Config.SW_Item"=w671) -> (w673:T47)
                  n320 = local write "SW Items"(w671) -> ()
                  n321 = local read "Station"() -> (w682:T4)
                  n322 = Bundle By Name(cluster=w682, "Name"=w681, "PN"=w680, "SN"=w679, "Location"=w678) -> (→"Station":T4)
                  n323 = Bundle By Name(cluster=w664, "RptHdr.Station"=w673, "Lists.DisableRouteCk"=w666) -> (w669:T73)
                }
                frame "Facility" {
                  n324 = Unbundle By Name(w688) -> ("CfgFilePaths.WorkingCfg"=w693:path)
                  n325 = Unbundle By Name(w688) -> ("RptHdr.Station.Name"=w686:string)
                  n326 = call "TestExec.Config, Get Facility Info.vi"("Facility Info"=w693) -> ("error out"=w691:errorcluster, "Facility Modes"=w684:path)  [unwired: 9 in]
                  n327 = call "Config.Read UUT Info.vi"("Default Process Step"=w686, "Default Product Name"="UNDEFINED", "Local Station Config File"=w693) -> ("error out"=w690:errorcluster, "Process Step"=w687:string, "Product"=w692:string)  [unwired: 6 in]
                  n328 = Bundle By Name(cluster=w688, "CfgFilePaths.ModeCfg"=w684, "Lists.Product"=w692, "Lists.ProcessStep"=w687, "RptHdr.Test Run.ProcessStep"=w687) -> (w694:T73)
                  n329 = Merge Errors(w691, w690) -> (w689:errorcluster)
                }
                frame "Barcode Input" {
                  n330 = Unbundle By Name(w700) -> ("Cfg.Dirs.Config"=w703:path)
                  n331 = Build Path(base path=w703, name or relative path="Barcode Config.ini") -> (appended path=w697:path)
                  n332 = call "TestExec.Config, Get Barcode PN SN Format Info.vi"("Config File"=w697) -> ("Barcode PN SN Format"=w702:T24)  [unwired: 9 in, 1 out]
                  n333 = local write "Barcode PN SN Format"(w702) -> ()
                }
                frame "Mode" {
                  # "Ignore error\nwill use default modes"
                  n334 = To Variant(anything=TRUE) -> (Variant=w714:variant)
                  n335 = call <vilib>:"Q.Enqueue Task.vi"("Data1"=w714, "Task Name"="Operator - Set Mode", "Q In"=w711) -> ()  [unwired: 7 in, 2 out]
                  n336 = Unbundle By Name(w710) -> ("ModeMgr"=w720:refnum<class "Mode Manager.lvclass">, "CfgFilePaths.ModeCfg"=w716:path)
                  n337 = control-ref of="Mode"() -> (w719:refnum<vi>)
                  n338 = call <vilib>:"Application Directory.vi"() -> ("Application Directory"=w706:path)
                  n339 = Build Path(base path=w706, name or relative path="Config\\Default Modes.json") -> (appended path=w704:path)
                  n340 = call "ModeMgr.Init.vi"("Default Config File"=w704, "ControlRef"=w719, "Config File"=w716, "ModeMgr In"=w720) -> ("error out"=w715:errorcluster, "Mode"=w717:string, "ModeMgr Out"=w718:refnum<class "Mode Manager.lvclass">)  [unwired: 4 in, 1 out]
                  n341 = call <vilib>:"Clear Errors.vi"("error in (no error)"=w715) -> ()  [unwired: 5 in, 2 out]
                  n342 = Bundle By Name(cluster=w710, "ModeMgr"=w718, "RptHdr.Test Run.Mode"=w717) -> (w709:T73)
                }
                frame "Route" {
                  # "Station Config has an item that points to a CSV file containing a list of routes.\nThe columns in the file are:\nCol0 = Route\nCol1 = StationName\n\nA list of routes \n\nEXAMPLE:\n[Routes]\nRouteList = \"C:\\MTE\\Facility\\Circle Test\\Circle Test Routes.csv\""
                  n343 = Unbundle By Name(w721) -> ("CfgFilePaths.WorkingCfg"=w727:path)
                  n344 = Unbundle By Name(w721) -> ("RptHdr.Station.Name"=w722:string)
                  n345 = call "TestExec.Get Route Config.vi"("Station Name"=w722, "Sta Config INI"=w727) -> ("Routes"=w726:string[])  [unwired: 7 in, 2 out]
                  n346 = Bundle By Name(cluster=w721, "Lists.UUTRoutes"=w726) -> (w725:T73)
                }
                frame "Sequences" {
                  n347 = Unbundle By Name(w729) -> ("CfgFilePaths.WorkingCfg"=w728:path)
                  n348 = Unbundle By Name(w732) -> ("Cfg.Dirs.Root"=w741:path)
                  n349 = call "TestExec.Get Sequence List.vi"("Working Config File"=w728, "Working Dir"=w741) -> ("error out"=w733:errorcluster, "Default Index"=w736:i32, "Sequences Info"=w738:T66[], "Seq Names"=w740:string[], "Repeat Delay"=w737:dbl, "AutoRepeat"=w735:bool)  [unwired: 4 in]
                  n350 = case shown="True" w735 {
                    tunnel: w734 -> [_ w745]
                    tunnel: w737 -> [_ w742]
                    frame False {
                    }
                    frame True {
                      w744 = TRUE ("Visible")
                      w746 = "Repeat Sequence - Auto" ("Sched Name")
                      n351 = Get Date/Time In Seconds() -> (seconds since 1Jan1904=w743:timestamp)
                      n352 = local write "Start Time"(w743) -> ()
                      n353 = local write "End Time"(w743) -> ()
                      n354 = call <vilib>:"Scheduler.AddTask.vi"("Interval(s)"=w742, "Task Name"=w746, "Sched Name"=w746, "Q In"=w745) -> ("Q Out"=w749:refnum<queue>)  [unwired: 6 in, 1 out]
                      n355 = property on="Repeat Notificaiton" class="Str"("Visible"=w744) -> ()  [unwired: 2 in, 2 out]
                      n356 = property on="Kill AutoLnch" class="Bool"("Visible"=w744) -> ()  [unwired: 2 in, 2 out]
                      n357 = call <vilib>:"Q.Enqueue Task.vi"("Top of Q"=TRUE, "Task Name"="Repeat Notification" ("Sched Name"), "Q In"=w749) -> ()  [unwired: 7 in, 2 out]
                    }
                  }
                  n358 = To Unsigned Word Integer(number=w736) -> (unsigned 16bit integer=w739:u16)
                  n359 = Bundle By Name(cluster=w729, "Sequences"=w738, "Repeat(s)"=w737, "Lists.Default Seq"=w736) -> (w731:T73)
                  n360 = property on="Sequence" class="Ring (strict)"("Strings []"=w740, "Value"=w739) -> ()  [unwired: 2 in, 2 out]
                }
                frame "Data Dir" {
                  n361 = Unbundle By Name(w754) -> ("Cfg.Dirs.Root"=w756:path)
                  n362 = Unbundle By Name(w759) -> ("CfgFilePaths.WorkingCfg"=w768:path)
                  n363 = Build Path(base path=w756, name or relative path="Data\\Local") -> (appended path=w755:path)
                  n364 = Bundle By Name(cluster=T23 {"Name"="Local Results", "Path"=path ""} ("Working Dirs"), "Name"="Local Results", "Path"=w755) -> (w751:T23)
                  n365 = Build Array(w751) -> (w752:T23[])
                  n366 = call "TestExec.Config, Read Test Data Dir Info.vi"("Dirs In"=w752, "Station Data Dir Config File"=w768) -> ("error out"=w769:errorcluster, "Working Dirs"=w750:T23[], "Seq Result Dirs"=w766:T23[])  [unwired: 5 in, 2 out]
                  n367 = Bundle By Name(cluster=T22 {"Station Data"=[], "SeqRsltDirs"=[]} ("Data Dir Config"), "Station Data"=w750, "SeqRsltDirs"=w766) -> (w767:T22)
                  "Data Dir Config" <- w767
                  n368 = case shown="Error" w769 {
                    selector: w769 -> [w771 w777]
                    tunnel: [w771 w776] -> w760
                    tunnel: w768 -> [_ w772]
                    frame No Error {
                    }
                    frame Error {
                      w773 = T74 -5201 items=["No Error"=0, "Abort"=-2, "Misc"=-5000, "Fixture Error"=-5100, "File IO - General"=-5200, "FIle IO - Config Error"=-5201, "Instrument - General"=-5300, "Instrument - Serial Com"=-5301, "Instrument - Camera"=-5302, "Instrument - PS"=-5303, "Instrument - Oscilloscope"=-5304, "Instrument - Function Gen"=-5305, "Instrument - Load"=-5306, "Instrument - Meter"=-5307, "Instrument - Power Control"=-5308, "Instrument - Motion"=-5309, "Instrument - RF"=-5310, "System Exe"=-5400, "Image Processing"=-5500, "Communication"=-5600, "Script - Syntax Error"=-6000, "Script - Invalid Name or Param"=-6100, "Script - Timeout"=-6200, "Invalid Data"=-6300, "FW Update Error"=-6500] ("Std Code")
                      n369 = Format Into String(format string="Error reading test station data directory config from \"%s\".", w772) -> (resulting string=w774:string)  [unwired: 2 in, 1 out]
                      n370 = call "Error.Set-Change Error Info.vi"("Std Code"=w773, "error in"=w777, "Description"=w774) -> ("error out"=w776:errorcluster)  [unwired: 8 in]
                    }
                  }
                  n371 = Bundle By Name(cluster=w759, "Data Dirs"=w767) -> (w758:T73)
                  n372 = Unbundle By Name(w758) -> ("Opts.DataDirEn"=w764:bool)
                  n373 = Current VI's Menubar() -> (w765:refnum<k9>)
                  n374 = call "TestExec.Add Data Folder Items to Menu.vi"("Working Dirs"=w750, "Enabled"=w764, "menu ref"=w765) -> ("error out"=w763:errorcluster)  [unwired: 8 in]
                  n375 = call <vilib>:"Clear Errors.vi"("error in (no error)"=w763) -> ()  [unwired: 5 in, 2 out]
                }
                frame "Misc Dirs" {
                  w787 = T74 -5201 items=["No Error"=0, "Abort"=-2, "Misc"=-5000, "Fixture Error"=-5100, "File IO - General"=-5200, "FIle IO - Config Error"=-5201, "Instrument - General"=-5300, "Instrument - Serial Com"=-5301, "Instrument - Camera"=-5302, "Instrument - PS"=-5303, "Instrument - Oscilloscope"=-5304, "Instrument - Function Gen"=-5305, "Instrument - Load"=-5306, "Instrument - Meter"=-5307, "Instrument - Power Control"=-5308, "Instrument - Motion"=-5309, "Instrument - RF"=-5310, "System Exe"=-5400, "Image Processing"=-5500, "Communication"=-5600, "Script - Syntax Error"=-6000, "Script - Invalid Name or Param"=-6100, "Script - Timeout"=-6200, "Invalid Data"=-6300, "FW Update Error"=-6500] ("Std Code")
                  w803 = T74 -5201 items=["No Error"=0, "Abort"=-2, "Misc"=-5000, "Fixture Error"=-5100, "File IO - General"=-5200, "FIle IO - Config Error"=-5201, "Instrument - General"=-5300, "Instrument - Serial Com"=-5301, "Instrument - Camera"=-5302, "Instrument - PS"=-5303, "Instrument - Oscilloscope"=-5304, "Instrument - Function Gen"=-5305, "Instrument - Load"=-5306, "Instrument - Meter"=-5307, "Instrument - Power Control"=-5308, "Instrument - Motion"=-5309, "Instrument - RF"=-5310, "System Exe"=-5400, "Image Processing"=-5500, "Communication"=-5600, "Script - Syntax Error"=-6000, "Script - Invalid Name or Param"=-6100, "Script - Timeout"=-6200, "Invalid Data"=-6300, "FW Update Error"=-6500] ("Std Code")
                  w804 = T74 -5201 items=["No Error"=0, "Abort"=-2, "Misc"=-5000, "Fixture Error"=-5100, "File IO - General"=-5200, "FIle IO - Config Error"=-5201, "Instrument - General"=-5300, "Instrument - Serial Com"=-5301, "Instrument - Camera"=-5302, "Instrument - PS"=-5303, "Instrument - Oscilloscope"=-5304, "Instrument - Function Gen"=-5305, "Instrument - Load"=-5306, "Instrument - Meter"=-5307, "Instrument - Power Control"=-5308, "Instrument - Motion"=-5309, "Instrument - RF"=-5310, "System Exe"=-5400, "Image Processing"=-5500, "Communication"=-5600, "Script - Syntax Error"=-6000, "Script - Invalid Name or Param"=-6100, "Script - Timeout"=-6200, "Invalid Data"=-6300, "FW Update Error"=-6500] ("Std Code")
                  n376 = Unbundle By Name(w782) -> ("CfgFilePaths.WorkingCfg"=w813:path, "Data Dirs.Station Data"=w812:T23[])
                  n377 = Unbundle By Name(w783) -> ("Cfg.Dirs.Root"=w811:path)
                  n378 = for {
                    tunnel: w812 -> [w821] mode=indexing
                    tunnel: [w820] -> w809
                    tunnel: [w817] -> w807
                    stop <- w820 stop-if-true
                    n379 = Unbundle By Name(w821) -> ("Path"=w817:path, "Name"=w819:string)
                    n380 = Equal?(x=w819, y="DataArchiveDir" ("x")) -> (x = y?=w820:bool)
                  }
                  n381 = Unbundle By Name(w783) -> ("Cfg.Dirs.Root"=w792:path)
                  n382 = Build Path(base path=w811, name or relative path="Data\\Archive") -> (appended path=w808:path)
                  n383 = Select(t=w807, s=w809, f=w808) -> (s? t:f=w779:path)
                  n384 = Build Path(base path=w792, name or relative path="Data\\Local") -> (appended path=w791:path)
                  n385 = call "TestExec.Config, Read ScriptSearchPaths.vi"("Station Data Dir Config File"=w813) -> ("error out"=w799:errorcluster, "ScriptSearchPaths"=w814:path[])  [unwired: 9 in]
                  n386 = call <vilib>:"File.Create Folder if Does Not Exist.vi"("Path"=w791) -> ("error out"=w785:errorcluster, "Dup Path"=w784:path)  [unwired: 8 in, 1 out]
                  n387 = To Variant(anything=w779) -> (Variant=w778:variant)
                  n388 = call <vilib>:"Q.Enqueue Task.vi"("Data1"=w778, "Q Name"="ArchiveMover", "Task Name"="SetArchiveDir" ("Q Name")) -> ()  [unwired: 7 in, 2 out]
                  n389 = call <vilib>:"File.Create Folder if Does Not Exist.vi"("Path"=w779) -> ("error out"=w798:errorcluster, "Dup Path"=w796:path)  [unwired: 8 in, 1 out]
                  n390 = Bundle By Name(cluster=w782, "CfgFilePaths.ScriptLibDirs"=w814, "CfgFilePaths.Archive"=w796, "CfgFilePaths.LocalData"=w784) -> (w815:T73)
                  n391 = Format Into String(format string="Error creating data archive dir.|Data Archive dir = \"%s\".", w796) -> (resulting string=w800:string)  [unwired: 2 in, 1 out]
                  n392 = Format Into String(format string="Error creating local data dir.|Local Data dir = \"%s\".", w784) -> (resulting string=w789:string)  [unwired: 2 in, 1 out]
                  n393 = call "Error.Set-Change Error Info.vi"("Std Code"=w803, "Append Details"=FALSE, "error in"=w798, "Description"=w800) -> ("error out"=w806:errorcluster)  [unwired: 7 in]
                  n394 = call "Error.Set-Change Error Info.vi"("Std Code"=w804, "Append Details"=FALSE, "error in"=w799, "Description"="Error reading script search dirs from config.") -> ("error out"=w805:errorcluster)  [unwired: 7 in]
                  n395 = call "Error.Set-Change Error Info.vi"("Std Code"=w787, "Append Details"=FALSE, "error in"=w785, "Description"=w789) -> ("error out"=w786:errorcluster)  [unwired: 7 in]
                  n396 = Merge Errors(w805, w806, w786) -> (w797:errorcluster)
                }
                frame "SW Check" {
                  n397 = call <vilib>:"Q.Enqueue Task.vi"("Task Name"="Get Released SW Files", "Q In"=w823) -> ()  [unwired: 8 in, 2 out]
                }
                frame "Done", Default {
                  n398 = Unbundle By Name(w838) -> ("Exe"=w837:bool)
                  n399 = Unbundle By Name(w831) -> ("Data Dirs.Station Data"=w833:T23[])
                  n400 = case shown="False" w837 {
                    tunnel: [w850 w854] -> w836
                    frame False {
                      n401 = control-ref of="This VI"() -> (w853:refnum<vi>)
                      n402 = property class="VI"(reference=w853) -> ("Path"=w852:path)  [unwired: 1 in, 2 out]
                      n403 = Build Path(base path=w852, name or relative path="..\\..\\..\\Common\\Utils\\Windows\\Devcon") -> (appended path=w850:path)
                    }
                    frame True {
                      n404 = call <vilib>:"Application Directory.vi"() -> ("Application Directory"=w856:path)
                      n405 = Build Path(base path=w856, name or relative path="Utils") -> (appended path=w854:path)
                    }
                  }
                  n406 = for {
                    tunnel: w833 -> [w849] mode=indexing
                    tunnel: [w846] -> w829
                    tunnel: [w845] -> w830
                    stop <- w845 stop-if-true
                    n407 = Unbundle By Name(w849) -> ("Path"=w846:path, "Name"=w847:string)
                    n408 = Equal?(x=w847, y="ResultsArchiveDir") -> (x = y?=w845:bool)
                  }
                  n409 = case shown="True" w830 {
                    tunnel: [w841 w844] -> w832
                    tunnel: w831 -> [w841 w843]
                    tunnel: w829 -> [_ w842]
                    frame False {
                    }
                    frame True {
                      n410 = Bundle By Name(cluster=w843, "CfgFilePaths.Archive"=w842) -> (w844:T73)
                    }
                  }
                  n411 = Build Path(base path=w836, name or relative path="Devcon.exe") -> (appended path=w834:path)
                  n412 = Bundle By Name(cluster=w832, "CfgFilePaths.Devcon"=w834) -> (w828:T73)
                  n413 = Unbundle By Name(w828) -> ("CfgFilePaths"=w827:T67)
                  n414 = local write "CfgFilePaths"(w827) -> ()
                }
              }
            }
            n415 = Merge Errors(w619) -> (w620:errorcluster)
          }
          frame "Config - Open Folder" {
            w862 = T23 {"Name"="Test Sequence Folder", "Path"=path ""} ("Working Dirs")
            n416 = Variant To Data(type="", Variant=w873) -> (data=w871:string)  [unwired: 1 in, 1 out]
            n417 = Unbundle By Name(w857) -> ("Cfg.Dirs.Root"=w867:path)
            n418 = Unbundle By Name(w857) -> ("Cfg.Dirs.Config"=w858:path)
            n419 = Build Path(base path=w867, name or relative path="Sequences" ("section")) -> (appended path=w865:path)
            n420 = Bundle By Name(cluster=w862, "Name"="Config Folder", "Path"=w858) -> (w861:T23)
            n421 = Bundle By Name(cluster=w862, "Name"="Test Sequence Folder", "Path"=w865) -> (w864:T23)
            n422 = Build Array(w861, w864) -> (w863:T23[])
            n423 = for {
              tunnel: w863 -> [w880] mode=indexing
              tunnel: [w879] -> w870
              tunnel: w871 -> [w877]
